vi "initWaves.vi"(8 "Microscope Settings":T1 {"Under Scan /ms" min=0.0 max=10.0 step=0.05; "ROI"."T"."Range /s" min=0.0 max=10.0 step=0.05; "ROI"."T"."Step /s" min=0.0 max=10.0 step=0.05; "ROI"."T"."Start /s" min=0.0 max=10.0 step=0.05; "ROI"."X"."Range /px" min=0.0 max=10.0 step=0.05; "ROI"."X"."Step /px" min=0.0 max=10.0 step=0.05; "ROI"."X"."Start /px" min=0.0 max=10.0 step=0.05; "ROI"."Y"."Range /px" min=0.0 max=10.0 step=0.05; "ROI"."Y"."Step /px" min=0.0 max=10.0 step=0.05; "ROI"."Y"."Start /px" min=0.0 max=10.0 step=0.05; "ROI"."Z"."Range /um" min=0.0 max=10.0 step=0.05; "ROI"."Z"."Step/um" min=0.0 max=10.0 step=0.05; "ROI"."Z"."Start /um" min=0.0 max=10.0 step=0.05; "Colour"."Filter" items=["Empty"=1, ""=2, ""=3, "561"=4, ""=5, "488"=6]; "Camera Delay /ms" min=0.0 max=10.0 step=0.05; "Trigger Source" items=["Internal"=1.0, "External"=2.0]; "Readout Direction" items=["Forward"=1.0, "Backward"=2.0]; "Slit"."Scanning Mode" items=["Full Frame"=1.0, "Slit Scanning"=12.0]; "Piezo Position /um" min=0.0 max=10.0 step=0.05}) -> (0 "Waveform Player":refnum<queue>, 1 "Digital":refnum<k21>, 2 "Analogue":refnum<k21>, 3 "Waveform Controller":refnum<queue>)   [LabVIEW 2015]
uses:
  controls/Microscope Settings.ctl
  controls/Hardware.ctl
  controls/ModeEnum.ctl
  controls/PinOut.ctl
  controls/PinOut2.ctl
  <vilib>/DAQmx/create/channels.llb/DAQmx Create Channel (DO-Digital Output).vi
  <vilib>/DAQmx/create/channels.llb/DAQmx Create Channel (AO-Voltage-Basic).vi
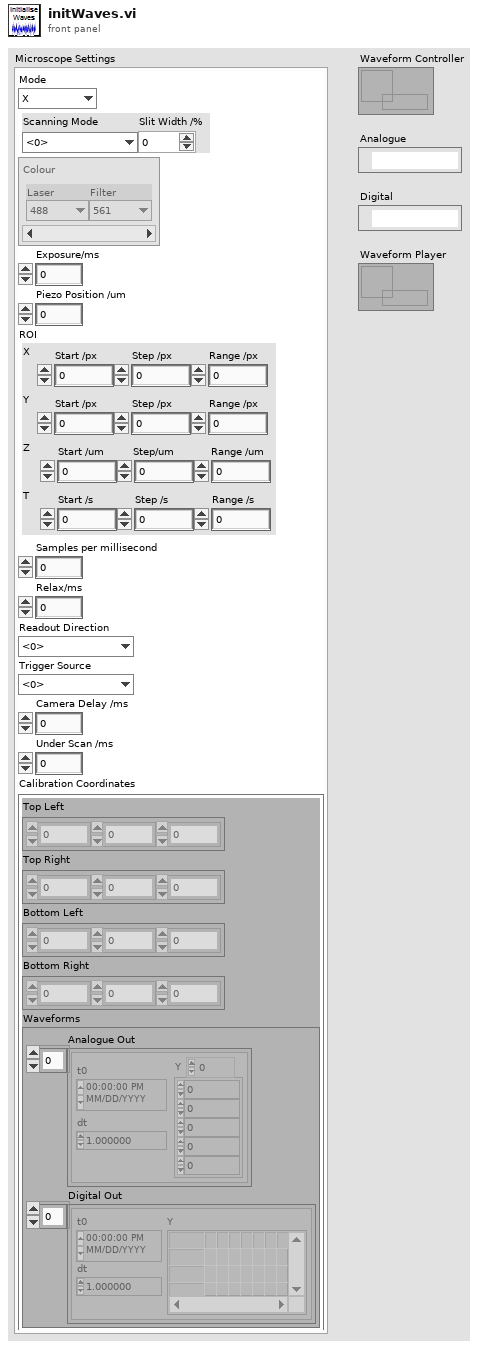
[diagram p1: front panel]
types:
  T1 = typedef "Microscope Settings.ctl" = cluster{"Mode":enum16{"X", "XY", "XYZ", "XYZT", "XYZC", "Tweezers", "Virus"}, "Slit":cluster{"Scanning Mode":dbl, "Slit Width /%":dbl}, "Colour":cluster{"Laser":enum16{"Brightfield", "445", "488", "561", "647"}, "Filter":u16}[], "Exposure/ms":dbl, "Piezo Position /um":dbl, "ROI":cluster{"X":cluster{"Start /px":dbl, "Step /px":dbl, "Range /px":dbl}, "Y":cluster{"Start /px":dbl, "Step /px":dbl, "Range /px":dbl}, "Z ":cluster{"Start /um":dbl, "Step/um":dbl, "Range /um":dbl}, "T ":cluster{"Start /s":dbl, "Step /s":dbl, "Range /s":dbl}}, "Samples per millisecond":dbl, "Relax/ms":dbl, "Readout Direction":dbl, "Trigger Source":dbl, "Camera Delay /ms":dbl, "Under Scan /ms":dbl, "Calibration Coordinates":cluster{"Top Left":dbl[], "Top Right":dbl[], "Bottom Left":dbl[], "Bottom Right":dbl[], "Waveforms":cluster{"Analogue Out":waveform(dbl)[], "Digital Out":digitalwaveform[]}}}
  T2 = typedef "Hardware.ctl" = enum16{"Stop", "RunCont", "EndCont", "Idle", "Update", "Run Waves"}
  T3 = typedef "ModeEnum.ctl" = enum16{"Idle", "generateWaves", "runWaves", "runWavesCont", "endWavesCont", "stop"}
  T4 = typedef "PinOut.ctl" = string
  T5 = typedef "PinOut2.ctl" = string
  T6 = cluster{"Analogue Out":waveform(dbl)[], "Digital Out":digitalwaveform[]}
  T7 = enum16{"X", "XY", "XYZ", "XYZT", "XYZC", "Tweezers", "Virus"}
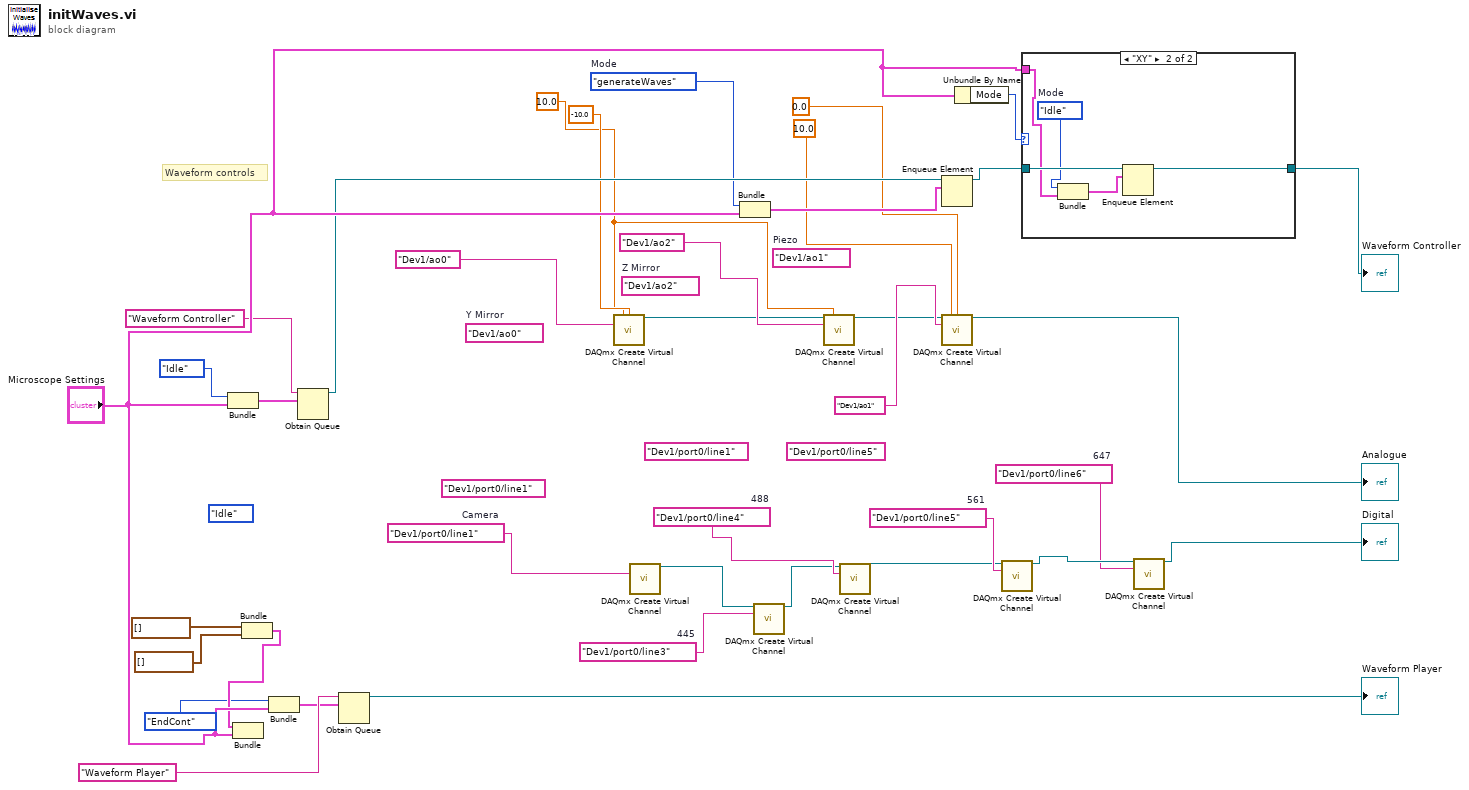
[diagram p0: block diagram]
diagram:
  (unwired) ModeEnum."Idle" ("Mode")
  w27 = tag "Dev1/port0/line6"  # 647
  w25 = tag "Dev1/port0/line5"  # 561
  w20 = tag "Dev1/port0/line3"  # 445
  (unwired) T4 "Dev1/port0/line1" ("Combo Box")
  (unwired) T5 "Dev1/port0/line1" ("Combo Box")
  (unwired) T4 "Dev1/port0/line5" ("Combo Box")
  w23 = tag "Dev1/port0/line4"  # 488
  w26 = tag "Dev1/port0/line1"  # Camera
  w8 = ModeEnum."generateWaves"  # Mode
  (unwired) tag "Dev1/ao1"  # Piezo
  (unwired) tag "Dev1/ao2"  # Z Mirror
  (unwired) tag "Dev1/ao0"  # Y Mirror
  w1 = 10.0 ("maximum value")
  # "Waveform controls"
  n1 = Bundle("Mode"=ModeEnum."Idle", "Microscope Settings"="Microscope Settings") -> (w10:cluster{"Mode":T3, "Microscope Settings":T1})  [unwired: 1 in]
  n2 = Bundle "Bundle"("Analogue Out"=waveform(dbl)[] [], "Digital Out"=digitalwaveform[] []) -> (w36:T6)  [unwired: 1 in]
  n3 = Bundle(w36, "Microscope Settings"="Microscope Settings") -> ()  [unwired: 1 in, 1 out]
  n4 = Bundle(Hardware."EndCont", "Microscope Settings"="Microscope Settings") -> (w30:cluster{T2, "Microscope Settings":T1})  [unwired: 1 in]
  n5 = Obtain Queue(name (unnamed)="Waveform Controller", element data type=w10) -> (queue out=w11:refnum<queue>)  [unwired: 3 in, 2 out]
  n6 = Obtain Queue(name (unnamed)="Waveform Player", element data type=w30) -> (queue out=→"Waveform Player":refnum<queue>)  [unwired: 3 in, 2 out]
  n7 = call-poly <vilib>:"DAQmx Create Virtual Channel.vi"("maximum value"=w1, "minimum value"=-10.0, "physical channels"=T4 "Dev1/ao0" ("Combo Box")) -> ("task out"=w6:refnum<k21>)  [unwired: 11 in, 1 out]
  n8 = call-poly <vilib>:"DAQmx Create Virtual Channel.vi"("lines"=w26) -> ("task out"=w21:refnum<k21>)  [unwired: 13 in, 1 out]
  n9 = Bundle("Mode"=w8, "Microscope Settings"="Microscope Settings") -> (w14:cluster{"Mode":T3, "Microscope Settings":T1})  [unwired: 1 in]
  n10 = call-poly <vilib>:"DAQmx Create Virtual Channel.vi"("task in"=w21, "lines"=w20) -> ("task out"=w22:refnum<k21>)  [unwired: 12 in, 1 out]
  n11 = call-poly <vilib>:"DAQmx Create Virtual Channel.vi"("task in"=w6, "maximum value"=w1, "physical channels"=T4 "Dev1/ao2" ("Combo Box")) -> ("task out"=w7:refnum<k21>)  [unwired: 11 in, 1 out]
  n12 = call-poly <vilib>:"DAQmx Create Virtual Channel.vi"("task in"=w22, "lines"=w23) -> ("task out"=w24:refnum<k21>)  [unwired: 12 in, 1 out]
  n13 = Enqueue Element(queue=w11, element=w14) -> (queue out=w13:refnum<queue>)  [unwired: 2 in, 2 out]
  n14 = call-poly <vilib>:"DAQmx Create Virtual Channel.vi"("task in"=w7, "maximum value"=10.0 ("minimum value"), "minimum value"=0.0 ("maximum value"), "physical channels"=T4 "Dev1/ao1" ("Combo Box")) -> ("task out"=→"Analogue":refnum<k21>)  [unwired: 10 in, 1 out]
  n15 = Unbundle By Name("Microscope Settings") -> ("Mode"=w15:T7)
  n16 = call-poly <vilib>:"DAQmx Create Virtual Channel.vi"("task in"=w24, "lines"=w25) -> ("task out"=w28:refnum<k21>)  [unwired: 12 in, 1 out]
  n17 = case shown="\"XY\"" w15 {
    tunnel: w13 -> [w38 w43]
    tunnel: "Microscope Settings" -> [_ w41]
    tunnel: [w38 w39] -> w16
    frame "X", Default {
    }
    frame "XY" {
      w40 = ModeEnum."Idle"  # Mode
      n18 = Bundle("Mode"=w40, "Microscope Settings"=w41) -> (w42:cluster{"Mode":T3, "Microscope Settings":T1})  [unwired: 1 in]
      n19 = Enqueue Element(queue=w43, element=w42) -> (queue out=w39:refnum<queue>)  [unwired: 2 in, 2 out]
    }
  }
  "Waveform Controller" <- w16
  n20 = call-poly <vilib>:"DAQmx Create Virtual Channel.vi"("task in"=w28, "lines"=w27) -> ("task out"=→"Digital":refnum<k21>)  [unwired: 12 in, 1 out]
